vi "Test 9 h6 to 66.vi"(8 "error in (no error)":errorcluster, 11 "Test Case In":refnum<class "Descrambler Test.lvclass">) -> (0 "error out":errorcluster, 3 "Test Case Out":refnum<class "Descrambler Test.lvclass">)   [LabVIEW 2020, in "Descrambler Test.lvclass"]
uses:
  Descrambler Test.lvclass
  C:/Program Files (x86)/National Instruments/LabVIEW 2020/vi.lib/Astemes/LUnit/Test Case.lvclass
  <vilib>/Astemes/LUnit/Test Case.lvclass/Test Case.ctl
  4993e8ee-a06a-463a-9684-69129f64d5ce.vi
  <vilib>/Astemes/LUnit/Append Pass Result.vi
  <vilib>/Astemes/LUnit/Append Fail Result.vi
  <vilib>/Astemes/LUnit/Describe Comparison.vi
  <vilib>/Astemes/LUnit/Compare Variants.vi
  <vilib>/Astemes/LUnit/Variant to string.vi
  <vilib>/Utility/Data Type/Get Type Information.vi
  <vilib>/Utility/LVClass/Get LV Class Name.vi
  Descrambler/Descrambler.lvclass
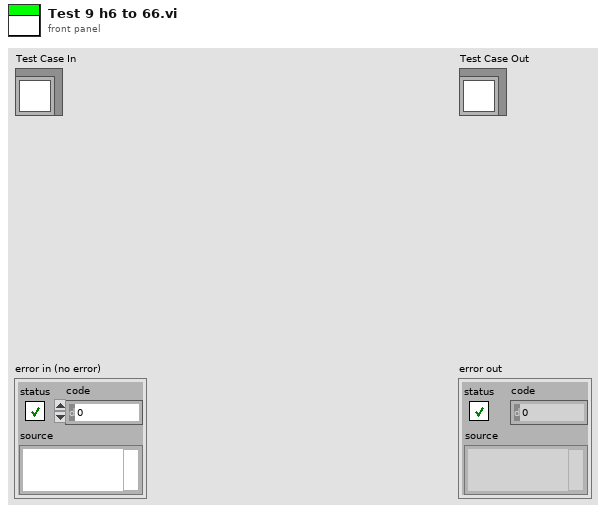
[diagram p1: front panel]
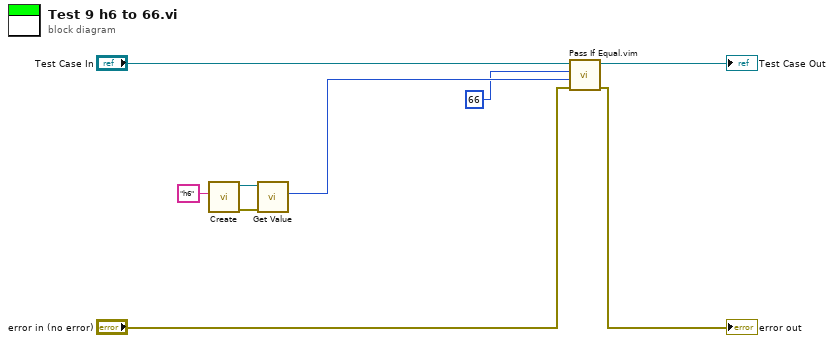
[diagram p0: block diagram]
diagram:
  n1 = call "Create.vi"("String"="h6") -> ("error out"=w4:errorcluster, "Descrambler"=w5:refnum<class "Descrambler.lvclass">)  [unwired: 9 in]
  n2 = call "Get Value.vi"("error in (no error)"=w4, "Descrambler in"=w5) -> ("Value"=w3:i32)  [unwired: 7 in, 2 out]
  n3 = call "Pass If Equal.vim"("error in (no error)"="error in (no error)", "Actual"=w3, "Expected"=66 ("Value"), "LUnit Test Case In"="Test Case In") -> ("error out"=→"error out":errorcluster, "LUnit Test Case Out"=→"Test Case Out":refnum<class "Descrambler Test.lvclass">)  [unwired: 6 in]
